vi "Disable stage.vi"(8 "error in (no error)":errorcluster, 11 "reference (out)":i32) -> (2 "X Pos":string, 3 "Y Pos":string)   [LabVIEW 2011]
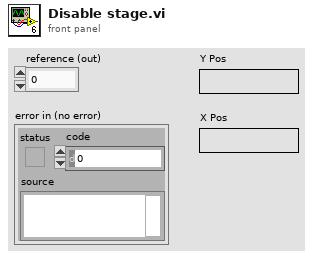
[diagram p1: front panel]
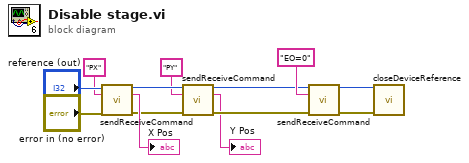
[diagram p0: block diagram]
diagram:
  n1 = call "sendReceiveCommand.vi"("reference (in)"="reference (out)", "write_string"="PX" ("raw_cmd"), "error in (no error)"="error in (no error)") -> ("reference (out)"=w3:i32, "read_string"=→"X Pos":string, "error out"=w2:errorcluster)  [unwired: 10 in]
  n2 = call "sendReceiveCommand.vi"("reference (in)"=w3, "write_string"="PY" ("raw_cmd"), "error in (no error)"=w2) -> ("reference (out)"=w8:i32, "read_string"=→"Y Pos":string, "error out"=w7:errorcluster)  [unwired: 10 in]
  n3 = call "sendReceiveCommand.vi"("reference (in)"=w8, "write_string"="EO=0" ("raw_cmd 2"), "error in (no error)"=w7) -> ("reference (out)"=w10:i32, "error out"=w9:errorcluster)  [unwired: 10 in, 1 out]
  n4 = call "closeDeviceReference.vi"("reference"=w10, "error in (no error)"=w9) -> ()  [unwired: 13 in, 1 out]
